vi "Read and Save as TDMS (Multiple Channels).vi"(0 "VISA resource name":refnum<visa-resource-name>, 1 "Segment Index (0)":i32 format="%.0g", 2 "TDMS Path":path, 5 "Measurement Source":i32[](array[ring])=[1, 2] items=["Channel 1"=1, "Channel 2"=2, "Channel 3"=3, "Channel 4"=4, "Function 1"=5, "Function 2"=6, "Function 3"=7, "Function 4"=8, "Memory 1"=9, "Memory 2"=10, "Memory 3"=11, "Memory 4"=12], 7 "Number of Samples (1000)":i32=1000, 9 "Maximum Time (10000ms)":u32=10000, 11 "error in (no error)":errorcluster, 12 "Offset (0)":i32, 13 "Waveform Format (0: Int8)":u16(ring) items=["Int8", "Int16", "Double"]) -> (4 "VISA resource name out":refnum<visa-resource-name>, 6 "Waveform Information":T1(array[cluster]), 10 "Written Samples":i32[](array[numeric]), 15 "error out":errorcluster)   [LabVIEW 2020, in "Agilent 90000 Series.lvlib"]
doc: "Returns scaled/unscaled data points of multiple channels from the instrument and save them into a TDMS file on the specified format."
uses:
  Agilent 90000 Series.lvlib
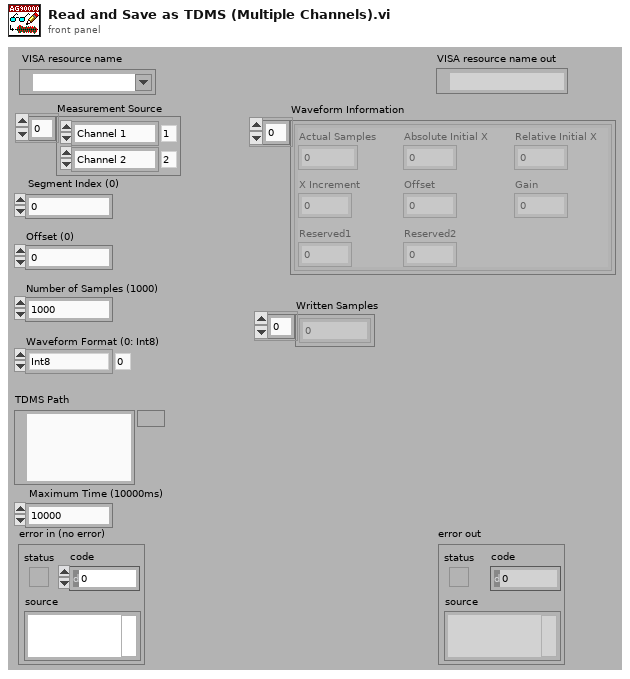
[diagram p1: front panel]
types:
  T1 = cluster{"Actual Samples":i32, "Absolute Initial X":dbl, "Relative Initial X":dbl, "X Increment":dbl, "Offset":dbl, "Gain":dbl, "Reserved1":dbl, "Reserved2":dbl}[]
  T2 = cluster{"Actual Samples":i32, "Absolute Initial X":dbl, "Relative Initial X":dbl, "X Increment":dbl, "Offset":dbl, "Gain":dbl, "Reserved1":dbl, "Reserved2":dbl}
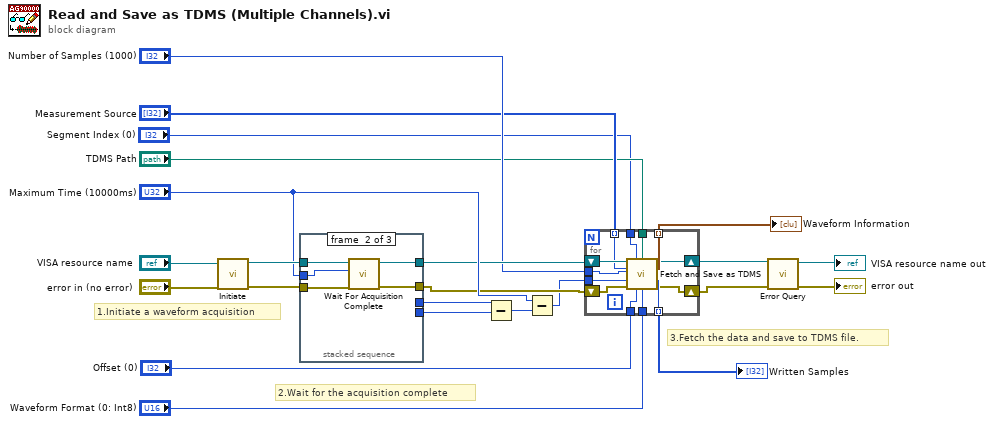
[diagram p0: block diagram]
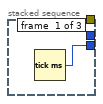
[diagram p2: hidden frame]
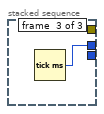
[diagram p3: hidden frame]
diagram:
  # "3.Fetch the data and save to TDMS file."
  # "2.Wait for the acquisition complete"
  # "1.Initiate a waveform acquisition"
  n1 = call "Initiate.vi"("error in (no error)"="error in (no error)", "VISA resource name"="VISA resource name") -> ("error out"=w20:errorcluster, "VISA resource name out"=w21:refnum<visa-resource-name>)  [unwired: 8 out]
  n2 = stacked-sequence {
    tunnel: [w24 _ _] -> w16
    tunnel: [_ _ w30] -> w17
    tunnel: w21 -> [_ w26 _]
    tunnel: [_ w29 _] -> w15
    tunnel: w20 -> [_ w27 _]
    tunnel: [_ w28 _] -> w14
    tunnel: "Maximum Time (10000ms)" -> [_ w25 _]
    frame #0 {
      n3 = Tick Count (ms)() -> (millisecond timer value=w24:u32)
    }
    frame #1 {
      n4 = call "Wait For Acquisition Complete.vi"("error in (no error)"=w27, "Maximum Time (10000ms)"=w25, "VISA resource name"=w26) -> ("error out"=w28:errorcluster, "VISA resource name out"=w29:refnum<visa-resource-name>)  [unwired: 7 out]
    }
    frame #2 {
      n5 = Tick Count (ms)() -> (millisecond timer value=w30:u32)
    }
  }
  n6 = Subtract(x=w17, y=w16) -> (x-y=w19:u32)
  n7 = Subtract(x="Maximum Time (10000ms)", y=w19) -> (x-y=w11:u32)
  n8 = for {
    tunnel: "Number of Samples (1000)" -> [w41]
    tunnel: "Measurement Source" -> [w40] mode=indexing
    tunnel: w11 -> [w39]
    tunnel: "TDMS Path" -> [w38]
    tunnel: [w37] -> w9 mode=indexing
    tunnel: [w36] -> w8 mode=indexing
    tunnel: "Offset (0)" -> [w33]
    tunnel: "Waveform Format (0: Int8)" -> [w32]
    tunnel: "Segment Index (0)" -> [w31]
    shift-right: [w35] -> w4
    shift-left: w15 -> [w43]
    shift-right: [w34] -> w1
    shift-left: w14 -> [w42]
    n9 = call "Fetch and Save as TDMS.vi"("VISA resource name"=w43, "Segment Index (0)"=w31, "TDMS Path"=w38, "Measurement Source (1: Channel 1)"=w40, "Number of Samples (1000)"=w41, "Maximum Time (10000ms)"=w39, "error in (no error)"=w42, "Offset (0)"=w33, "Waveform Format (0: Int8)"=w32) -> ("VISA resource name out"=w35:refnum<visa-resource-name>, "Waveform Information"=w37:T2, "Written Samples"=w36:i32, "error out"=w34:errorcluster)  [unwired: 3 out]
  }
  "Waveform Information" <- w9
  "Written Samples" <- w8
  n10 = call "Error Query.vi"("error in (no error)"=w1, "VISA resource name"=w4) -> ("error out"=→"error out":errorcluster, "VISA resource name out"=→"VISA resource name out":refnum<visa-resource-name>)  [unwired: 8 out]
